vi "Write Distance Gauge.vi"(10 "Distance Gauge":T1={"Serial"={"Serial Protocol"=enum."RS485", "Protocol Parameters"={"VISA resource name"="", "Baud Rate"=9600, "Data Bits"=8, "Parity"=enum."None", "Flow Control"=0, "Stop Bits"=10, "Timeout (ms)"=10000}, "Serial Message Parameters"={"Byte Count"=200, "Enable Termination Character"=FALSE, "Termination Char"=200}}, "Channels To Read"=[]} {"Serial"."Serial Message Parameters"."Termination Char" format="%x"; "Serial"."Protocol Parameters"."Stop Bits" items=["1.0"=10, "1.5"=15, "2.0"=20]; "Serial"."Protocol Parameters"."Flow Control" items=["None", "XON/XOFF", "RTS/CTS", "XON/XOFF & RTS/CTS", "DTR/DSR", "XON/XOFF & DTR/DSR"]; "Serial"."Protocol Parameters"."Data Bits" min=5 max=8 step=1}, 11 "DistanceGauge in":refnum<class "DistanceGauge.lvclass">) -> (3 "DistanceGauge out":refnum<class "DistanceGauge.lvclass">)   [LabVIEW 2013, in "DistanceGauge.lvlib" / "DistanceGauge.lvclass"]
uses:
  <userlib>/Common/Devices/DistanceGauge/DistanceGauge/DistanceGauge.lvclass
  <userlib>/Common/Devices/DistanceGauge/Config/Distance Gauge.ctl
  <userlib>/Common/SerialProtocols/Configuration/SerialConfig.ctl
  <userlib>/Common/SerialProtocols/Configuration/SerialProtocol.ctl
  <userlib>/Common/SerialProtocols/Configuration/ProtocolParameters.ctl
  <userlib>/Common/SerialProtocols/Configuration/SerialMessageParameters.ctl
  <userlib>/Common/Devices/DistanceGauge/Config/ChannelsToRead.ctl
  <userlib>/Common/Devices/DistanceGauge/DistanceGauge/DistanceGauge.lvclass/DistanceGauge.ctl
  <userlib>/Common/SerialProtocols/SerialProtocols.lvlib
  <userlib>/Common/Devices/DistanceGauge/DistanceGauge.lvlib
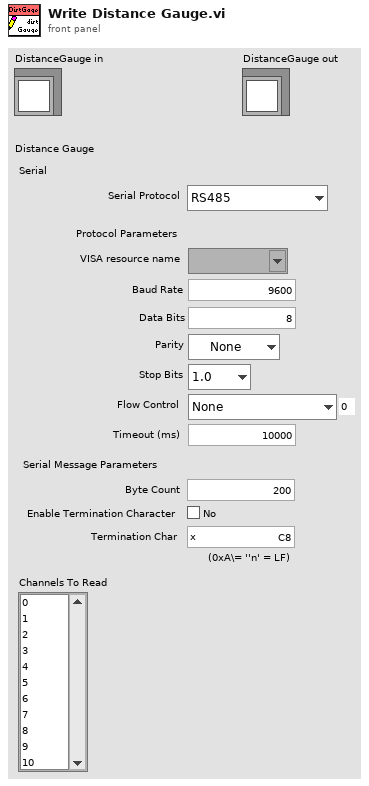
[diagram p1: front panel]
types:
  T1 = typedef "DistanceGauge.lvlib/Distance Gauge.ctl" = cluster{"Serial":T2, "Channels To Read":T6}
  T2 = typedef "SerialProtocols.lvlib/SerialConfig.ctl" = cluster{"Serial Protocol":T3, "Protocol Parameters":T4, "Serial Message Parameters":T5}
  T3 = typedef "SerialProtocols.lvlib/SerialProtocol.ctl" = enum16{"RS232", "RS485", "SerialSimulator"}
  T4 = typedef "SerialProtocols.lvlib/ProtocolParameters.ctl" = cluster{"VISA resource name":refnum<visa-resource-name>, "Baud Rate":u32, "Data Bits":u16, "Parity":enum16{"None", "Odd", "Even", "Mark", "Space"}, "Flow Control":u16, "Stop Bits":u16, "Timeout (ms)":u32}
  T5 = typedef "SerialProtocols.lvlib/SerialMessageParameters.ctl" = cluster{"Byte Count":u32, "Enable Termination Character":bool, "Termination Char":u8}
  T6 = typedef "DistanceGauge.lvlib/ChannelsToRead.ctl" = i32[]
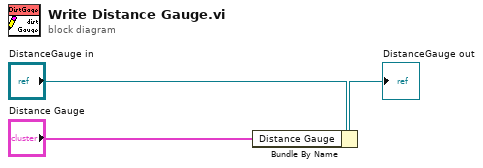
[diagram p0: block diagram]
diagram:
  n1 = Bundle By Name(cluster="DistanceGauge in", "Distance Gauge"="Distance Gauge") -> (→"DistanceGauge out":refnum<class "DistanceGauge.lvclass">)
